vi "addToList.vi"(8 "error in (no error)":errorcluster, 9 "CompiledScript":T1, 10 "Path":path, 11 "CompiledList in":refnum<class "CompiledList.lvclass">) -> (0 "error out":errorcluster, 3 "CompiledList out":refnum<class "CompiledList.lvclass">)   [LabVIEW 2011, in "Compiler.lvlib" / "CompiledList.lvclass"]
uses:
  CompiledList.lvclass
  ScriptListCompiler/ScriptListCompiler.lvclass
  Hal/Channels/VoltOutput/AnalogOutput.lvclass
  Hal/Channels/Digital/DigitalOutput.lvclass
  Hal/Channels/DDSOutput/Generic/DDSOutput.lvclass
  CompiledList.lvclass/CompiledList.ctl
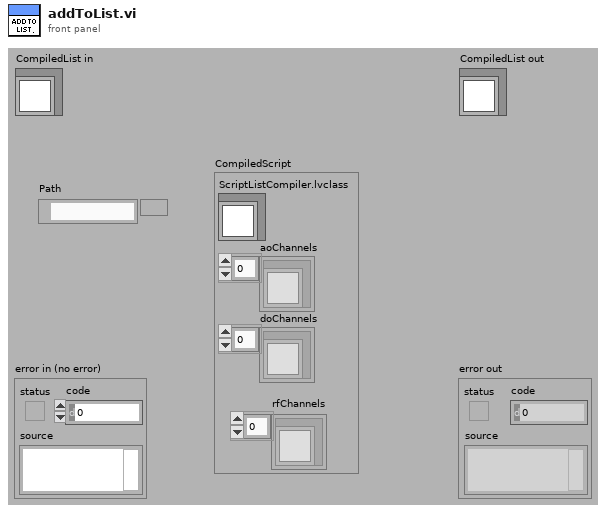
[diagram p1: front panel]
types:
  T1 = cluster{"ScriptListCompiler.lvclass":refnum<class "ScriptListCompiler.lvclass">, "aoChannels":refnum<class "AnalogOutput.lvclass">[], "doChannels":refnum<class "DigitalOutput.lvclass">[], "rfChannels":refnum<class "DDSOutput.lvclass">[]}
  T2 = cluster{"ScriptListCompiler.lvclass":refnum<class "ScriptListCompiler.lvclass">, "aoChannels":refnum<class "AnalogOutput.lvclass">[], "doChannels":refnum<class "DigitalOutput.lvclass">[], "rfChannels":refnum<class "DDSOutput.lvclass">[]}[]
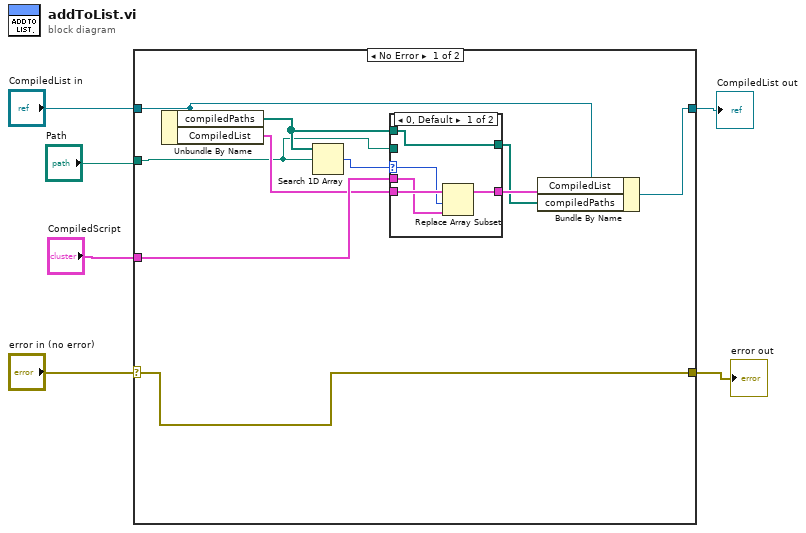
[diagram p0: block diagram]
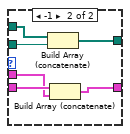
[diagram p2: hidden frame]
diagram:
  n1 = case shown="No Error" "error in (no error)" {
    selector: "error in (no error)" -> [w16 w29]
    tunnel: [w16 w29] -> w5
    tunnel: [w12 w28] -> w3
    tunnel: "CompiledList in" -> [w13 w28]
    tunnel: "Path" -> [w8 _]
    tunnel: "CompiledScript" -> [w15 _]
    frame No Error {
      n2 = Unbundle By Name(w13) -> ("compiledPaths"=w9:path[], "CompiledList"=w11:T2)
      n3 = Search 1D Array(1D array=w9, element=w8) -> (index of element=w10:i32)  [unwired: 1 in]
      n4 = case shown="0, Default" w10 {
        selector: w10 -> [w18 _]
        tunnel: [w17 w25] -> w14
        tunnel: w11 -> [w20 w27]
        tunnel: w15 -> [w19 w26]
        tunnel: w9 -> [w21 w24]
        tunnel: w8 -> [_ w23]
        tunnel: [w21 w22] -> w7
        frame 0, Default {
          n5 = Replace Array Subset(array=w20, new element=w19, index=w18) -> (w17:T2)
        }
        frame -1 {
          n6 = Build Array (concatenate)(w24, w23) -> (w22:path[])
          n7 = Build Array (concatenate)(w27, w26) -> (w25:T2)
        }
      }
      n8 = Bundle By Name(cluster=w13, "CompiledList"=w14, "compiledPaths"=w7) -> (w12:refnum<class "CompiledList.lvclass">)
    }
    frame Error {
    }
  }
  "error out" <- w5
  "CompiledList out" <- w3
